vi "FILE Write.vi"(0 "File Path (dialog if empty)":path, 1 "Start Path":path, 2 "Delimiter (Tab)":string="\t", 3 "Pattern":string, 5 "Spreadsheet Data":string[][](array[string]), 7 "Write String":string, 9 "File Type (Text)":T4, 11 "Error In (no error)":errorcluster, 12 "Append/Overwrite (Overwrite)":T3, 13 "New Line on Append?":T2, 14 "Warn on Overwrite (Warn)":T1) -> (4 "New File Path":path, 15 "Error Out":errorcluster)   [LabVIEW 2011]
doc: "This VI writes data to a file. File Open and File Close operations are also handled here.\n\nspreadsheed file? : controls if the 2D array input should be used to write a spreadsheet file, or the 'write string' should be used for writing a normal text file.\n\nnew line on append? : controls the insertion of a new line before the append in append mode. [\\r\\n] is used for a new line.\n\nappend mode: controls the mode that the write operation will take if the file path already exhists. If append is selected then the text (or spreadsheed array) will be appended to the data after the last character in the file. If overwrite is selected then the file will be overwritten by the new data specified.\n\nwarning dialog mode : controls the action of the dialog to warn when a file is about to be overwritten. If 'don't warn' is selected then the file will be automatically overwritten. If the dialog appears and the user chooses not to overwrite then no file operation will take place and no errors will ocurr.\n\nnote: generally canceling out of all dialog boxes will not cause a file error to ocurr, only actual file errors will be flagged."
uses:
  Type Defs/FILE Type Enum.ctl
  Type Defs/FILE Append Mode Enum.ctl
  Type Defs/FILE New Line Enum.ctl
  Type Defs/FILE Overwrite Warning Enum.ctl
panel:
  in  "Default Name":string
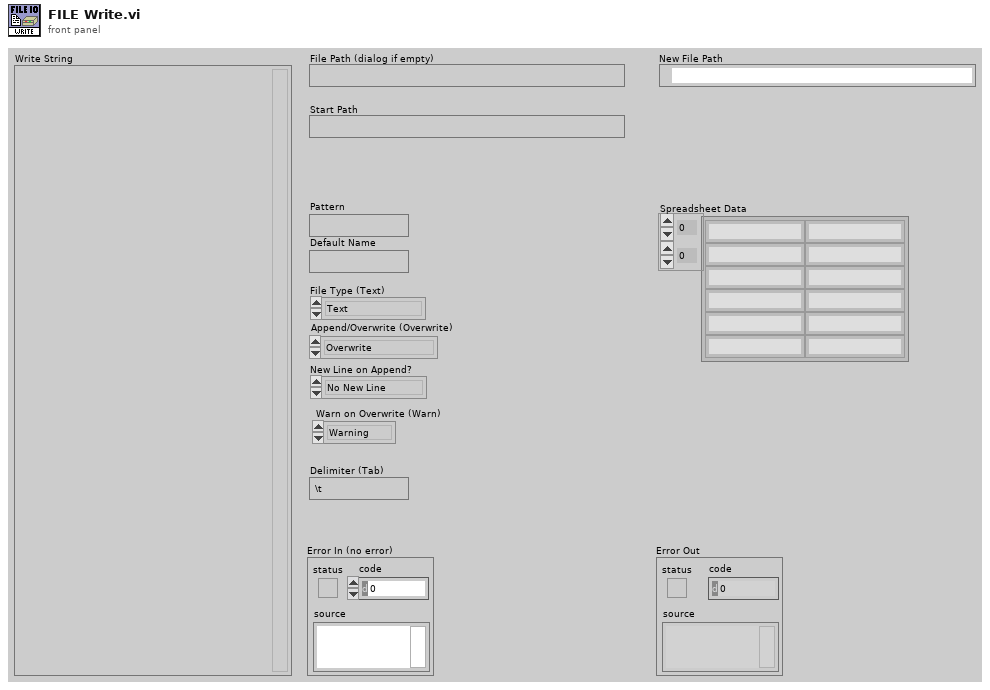
[diagram p1: front panel]
types:
  T1 = typedef "FILE Overwrite Warning Enum.ctl" = enum16{"Warning", "No Warning"}
  T2 = typedef "FILE New Line Enum.ctl" = enum16{"No New Line", "New Line"}
  T3 = typedef "FILE Append Mode Enum.ctl" = enum16{"Overwrite", "Append"}
  T4 = typedef "FILE Type Enum.ctl" = enum16{"Text", "Spreadsheet"}
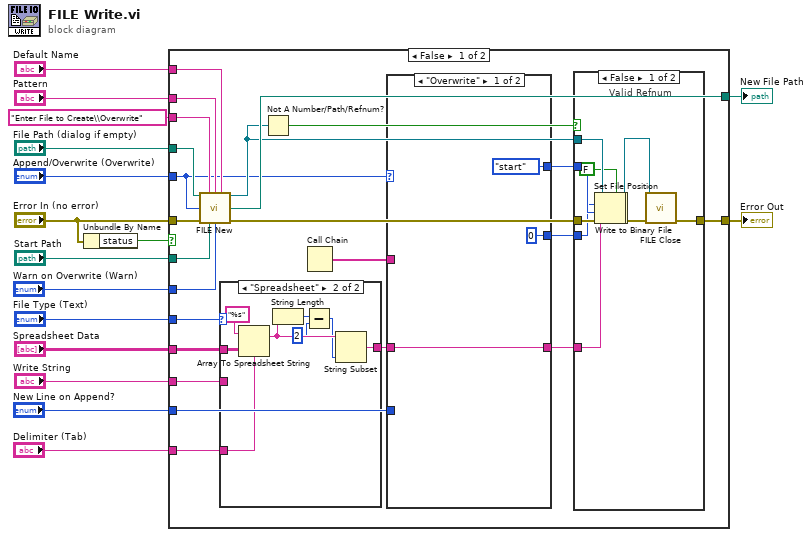
[diagram p0: block diagram]
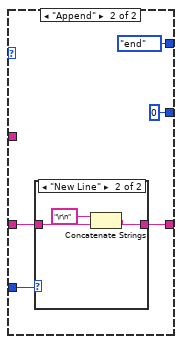
[diagram p2: hidden frame]
diagram:
  n1 = Unbundle By Name("Error In (no error)") -> ("status"=w11:bool)
  n2 = case shown="False" w11 {
    tunnel: [w39 w73] -> w12
    tunnel: "Error In (no error)" -> [w38 w73]
    tunnel: [w35 path ""] -> w14
    tunnel: "Enter File to Create\\Overwrite" ("prompt") -> [w36 _]
    tunnel: "File Path (dialog if empty)" -> [w37 _]
    tunnel: "Append/Overwrite (Overwrite)" -> [w26 _]
    tunnel: "Spreadsheet Data" -> [w33 _]
    tunnel: "File Type (Text)" -> [w34 _]
    tunnel: "Write String" -> [w32 _]
    tunnel: "Start Path" -> [w31 _]
    tunnel: "Pattern" -> [w30 _]
    tunnel: "Default Name" -> [w29 _]
    tunnel: "New Line on Append?" -> [w22 _]
    tunnel: "Warn on Overwrite (Warn)" -> [w20 _]
    tunnel: "Delimiter (Tab)" -> [w19 _]
    frame False {
      n3 = call "FILE New.vi"("New File Path"=w37, "Prompt"=w36, "Pattern"=w30, "Default Name"=w29, "Append Mode (Overwrite)"=w26, "Error In (no error)"=w38, "Start Path"=w31, "Warn on Overwrite (warn)"=w20) -> ("Refnum"=w28:refnum<file>, "File Path"=w35:path, "Error Out"=w18:errorcluster)  [unwired: 5 out]
      n4 = case shown="\"Spreadsheet\"" w34 {
        tunnel: w33 -> [_ w72]
        tunnel: [w64 w66] -> w23
        tunnel: w32 -> [w64 _]
        tunnel: w19 -> [_ w65]
        frame "Text" {
        }
        frame "Spreadsheet" {
          n5 = Array To Spreadsheet String(delimiter (Tab)=w65, array=w72, 3:"%s" ("format string")) -> (spreadsheet string=w70:string)
          n6 = String Length(string=w70) -> (length=w69:i32)
          n7 = Subtract(x=w69, y=2) -> (x-y=w67:i32)
          n8 = String Subset(string=w70, length (rest)=w67) -> (substring=w66:string)  [unwired: 1 out]
        }
      }
      n9 = Not A Number/Path/Refnum?(number/path/refnum=w28) -> (NaN/Path/Refnum?=w27:bool)
      n10 = Call Chain() -> (call chain=w17:string[])
      n11 = case shown="\"Overwrite\"" w26 {
        tunnel: [enum16{"start", "end", "current"}."start" ("pos mode (0:2)") enum16{"start", "end", "current"}."end" ("pos mode (0:2)")] -> w25
        tunnel: [0 ("pos offset (0)") 0 ("pos offset (0)")] -> w24
        tunnel: w23 -> [w40 w45]
        tunnel: w22 -> [_ w44]
        tunnel: [w40 w43] -> w21
        tunnel: w17 -> [_ _]
        frame "Overwrite" {
        }
        frame "Append" {
          n12 = case shown="\"New Line\"" w44 {
            tunnel: w45 -> [w48 w49]
            tunnel: [w48 w51] -> w43
            frame "No New Line" {
            }
            frame "New Line" {
              n13 = Concatenate Strings("\r\n", w49) -> (w51:string)
            }
          }
        }
      }
      n14 = case shown="False" w27 {
        tunnel: w28 -> [w62 _]
        tunnel: w18 -> [w61 w63]
        tunnel: [w58 w63] -> w39
        tunnel: w25 -> [w57 _]
        tunnel: w24 -> [w56 _]
        tunnel: w21 -> [w55 _]
        frame False {
          # "Valid Refnum"
          n15 = Set File Position(offset (in bytes) (0)=w56, refnum=w62, from (0:start)=w57, error in=w61) -> (refnum out=w54:refnum<file>, error out=w53:errorcluster)
          n16 = Write to Binary File(file (use dialog)=w54, data=w55, error in=w53, 5:FALSE ("prepend array or string size? (T)")) -> (refnum out=w59:refnum<file>, error out=w60:errorcluster)  [unwired: 3 out]
          n17 = call "FILE Close.vi"("Error In (no error)"=w60, "Refnum"=w59) -> ("Error Out"=w58:errorcluster)  [unwired: 5 out]
        }
        frame True {
          # "Invalid Refnum"
        }
      }
    }
    frame True {
      (unwired) ""
    }
  }
  "New File Path" <- w14
  "Error Out" <- w12
